vi "get_step.vi"(8 "error in (no error)":errorcluster, 11 "DL090409StageScaffold in":refnum<class "StageDL090409Scaffold.lvclass">) -> (0 "error out":errorcluster, 2 "step vector":refnum<class "SpaceVector.lvclass">, 3 "DL090409StageScaffold out":refnum<class "StageDL090409Scaffold.lvclass">)   [LabVIEW 2010, in "StageDL090409Scaffold.lvclass"]
uses:
  StageDL090409Scaffold.lvclass
  common/classes/SpaceVector/SpaceVector/SpaceVector.lvclass
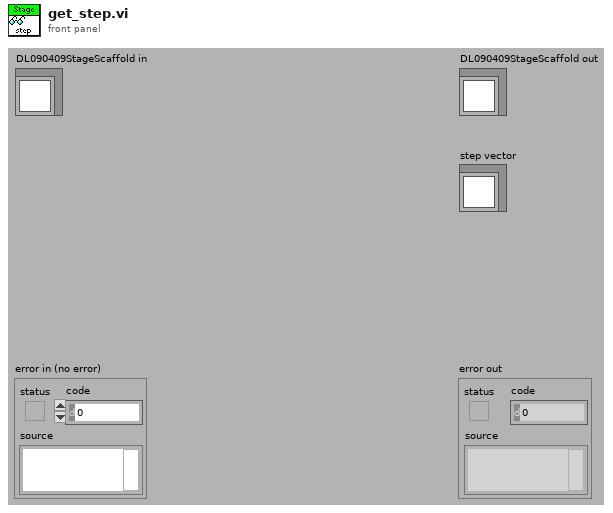
[diagram p1: front panel]
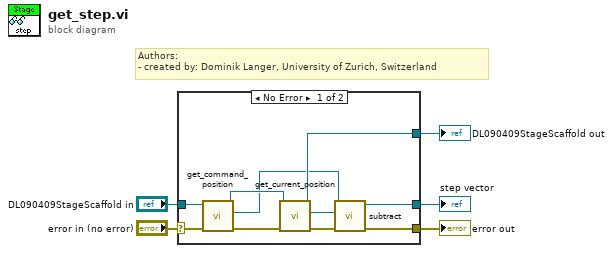
[diagram p0: block diagram]
diagram:
  # "Authors: \n- created by: Dominik Langer, University of Zurich, Switzerland"
  n1 = case shown="No Error" "error in (no error)" {
    selector: "error in (no error)" -> [w14 w17]
    tunnel: [w8 w17] -> w4
    tunnel: [w11 w16] -> w2
    tunnel: "DL090409StageScaffold in" -> [w12 w16]
    tunnel: [w6 _] -> w1
    frame No Error {
      n2 = call-dynamic "get_command_position.vi"("error in (no error)"=w14, "DL090409StageScaffold.lvclass in"=w12) -> ("error out"=w15:errorcluster, "SpaceVector.lvclass"=w10:refnum<class "SpaceVector.lvclass">, "DL090409StageScaffold.lvclass out"=w13:refnum<class "StageDL090409Scaffold.lvclass">)  [unwired: 7 out]
      n3 = call-dynamic "get_current_position.vi"("error in (no error)"=w15, "DL090409StageScaffold.lvclass in"=w13) -> ("error out"=w9:errorcluster, "current position"=w7:refnum<class "SpaceVector.lvclass">, "DL090409StageScaffold.lvclass out"=w11:refnum<class "StageDL090409Scaffold.lvclass">)  [unwired: 7 out]
      n4 = call "subtract.vi"("error in (no error)"=w9, "subtrahend"=w7, "SpaceVector in"=w10) -> ("error out"=w8:errorcluster, "SpaceVector out"=w6:refnum<class "SpaceVector.lvclass">)  [unwired: 7 out]
    }
    frame Error {
    }
  }
  "error out" <- w4
  "DL090409StageScaffold out" <- w2
  "step vector" <- w1
